vi "ExtractChannel.vi"(6 "Analytes":string[](array[string]), 9 "DataPile":T1(array[cluster]), 10 "dt":dbl, 11 "Channel":string) -> (3 "Graphs":cluster{dbl[], dbl[]}[](array[cluster]))   [LabVIEW 2024]
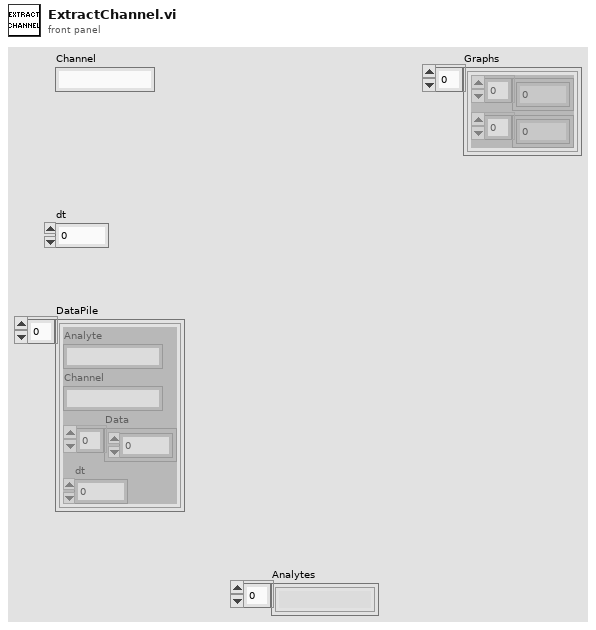
[diagram p1: front panel]
types:
  T1 = cluster{"Analyte":string, "Channel":string, "Data":dbl[], "dt":dbl}[]
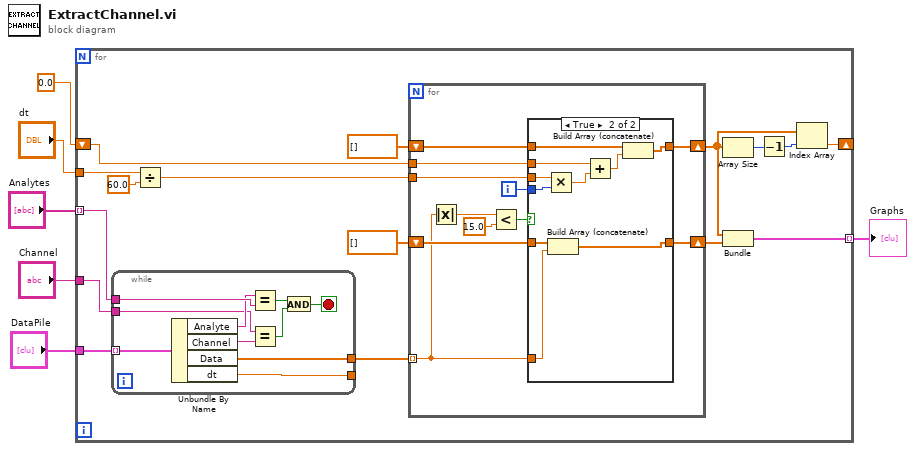
[diagram p0: block diagram]
diagram:
  n1 = for {
    tunnel: "Analytes" -> [w22] mode=indexing
    tunnel: "Channel" -> [w21]
    shift-right: [w10] -> _
    shift-left: 0.0 -> [w20]
    tunnel: [w18] -> w3 mode=indexing
    tunnel: "DataPile" -> [w8]
    tunnel: "dt" -> [w7]
    n2 = while {
      tunnel: w8 -> [w55] mode=indexing
      tunnel: w22 -> [w54]
      tunnel: w21 -> [w51]
      tunnel: [w47] -> w19
      tunnel: [w46] -> _
      stop <- w48 stop-if-true
      n3 = Unbundle By Name(w55) -> ("Analyte"=w53:string, "Channel"=w52:string, "Data"=w47:dbl[], "dt"=w46:dbl)
      n4 = Equal?(x=w53, y=w54) -> (x = y?=w50:bool)
      n5 = Equal?(x=w51, y=w52) -> (x = y?=w49:bool)
      n6 = And(x=w50, y=w49) -> (x .and. y?=w48:bool)
    }
    n7 = Divide(x=w7, y=60.0) -> (x/y=w16:dbl)
    n8 = for {
      tunnel: w19 -> [w27] mode=indexing
      shift-right: [w33] -> w12
      shift-left: dbl[] [] -> [w30]
      tunnel: w16 -> [w32]
      tunnel: w20 -> [w31]
      shift-right: [w29] -> w9
      shift-left: dbl[] [] -> [w28]
      i -> [w26]
      n9 = Absolute Value(x=w27) -> (abs(x)=w24:dbl)
      n10 = Less?(x=w24, y=15.0) -> (x < y?=w23:bool)
      n11 = case shown="True" w23 {
        tunnel: [w35 w45] -> w33
        tunnel: w26 -> [_ w44]
        tunnel: w32 -> [_ w42]
        tunnel: w31 -> [_ w41]
        tunnel: w30 -> [w35 w40]
        tunnel: [w34 w39] -> w29
        tunnel: w28 -> [w34 w38]
        tunnel: w27 -> [_ w37]
        frame False {
        }
        frame True {
          n12 = Multiply(x=w42, y=w44) -> (x*y=w43:dbl)
          n13 = Build Array (concatenate)(w38, w37) -> (w39:dbl[])
          n14 = Add(x=w41, y=w43) -> (x+y=w36:dbl)
          n15 = Build Array (concatenate)(w40, w36) -> (w45:dbl[])
        }
      }
    }
    n16 = Array Size(array=w12) -> (size(s)=w13:i32)
    n17 = Bundle(w12, w9) -> (w18:cluster{dbl[], dbl[]})  [unwired: 1 in]
    n18 = Decrement(x=w13) -> (x-1=w11:i32)
    n19 = Index Array(array=w12, index=w11) -> (element=w10:dbl)
  }
  "Graphs" <- w3
